vi "DeviceConfigurationState.vi"(5 "error out":errorcluster) -> (14 "image":i32[][](array[numeric]), 19 "error out 2":errorcluster)   [LabVIEW 2011]
uses:
  Variables/GlobalGetConfigurationStatus.vi
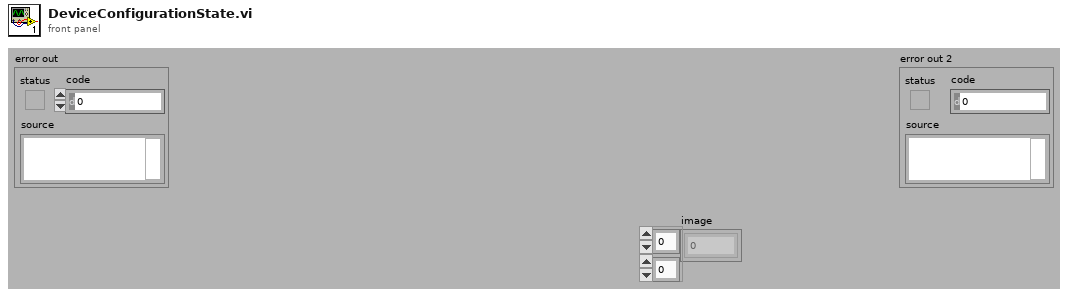
[diagram p1: front panel]
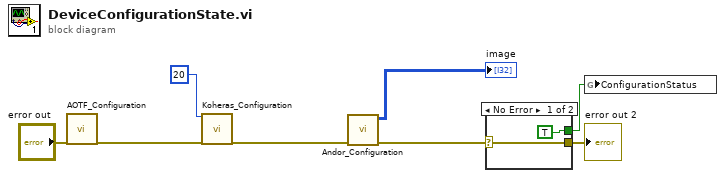
[diagram p0: block diagram]
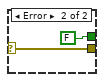
[diagram p2: hidden frame]
diagram:
  n1 = call "AOTF_Configuration.vi"("error out"="error out") -> ("error out 2"=w6:errorcluster)  [unwired: 18 in]
  n2 = call "Koheras_Configuration.vi"("laserPower"=20, "error in"=w6) -> ("out"=w5:errorcluster)  [unwired: 17 in]
  n3 = call "Andor_Configuration.vi"("Error in"=w5) -> ("error out"=w3:errorcluster, "image"=→"image":i32[][])  [unwired: 9 in]
  n4 = case shown="No Error" w3 {
    selector: w3 -> [w9 w12]
    tunnel: [w9 w12] -> w8
    tunnel: [TRUE ("ConfigurationStatus") FALSE ("ConfigurationStatus")] -> w7
    frame No Error {
    }
    frame Error {
    }
  }
  "error out 2" <- w8
  n5 = global write "GlobalGetConfigurationStatus.vi" "ConfigurationStatus"(w7) -> ()
